vi "sib vi - cycle fail v1.vi"(0 "Amps Lo?":bool, 1 "Enable in":bool, 2 "Input Cluster":T1, 3 "SELECT":T2(ring), 4 "Amps Hi?":bool) -> (14 "(FAIL LO) out":dbl, 15 "(FAIL HI) out":dbl, 16 "(DISP) out":T3, 17 "(RESULT) out":bool, 19 "file error":errorcluster)   [LabVIEW 2013]
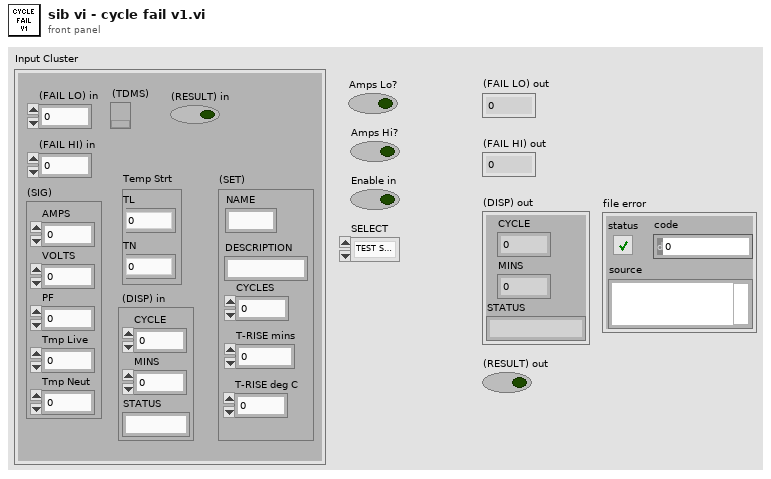
[diagram p1: front panel]
types:
  T1 = cluster{"(FAIL LO) in":dbl, "(FAIL HI) in":dbl, "(SIG)":cluster{"AMPS":dbl, "VOLTS":dbl, "PF":dbl, "Tmp Live":dbl, "Tmp Neut":dbl}, "Temp Strt":cluster{"TL":dbl, "TN":dbl}, "(SET)":cluster{"NAME":string, "DESCRIPTION":string, "CYCLES":dbl, "T-RISE mins":dbl, "T-RISE deg C":dbl}, "(TDMS)":refnum<k34>, " (DISP) in":cluster{"CYCLE":dbl, "MINS":dbl, "STATUS":string}, "(RESULT) in":bool}
  T2 = enum32{"TEST SET UP", "CYCLE TEST", "T-RISE TEST"}
  T3 = cluster{"CYCLE":dbl, "MINS":dbl, "STATUS":string}
  T4 = cluster{"AMPS":dbl, "VOLTS":dbl, "PF":dbl, "Tmp Live":dbl, "Tmp Neut":dbl}
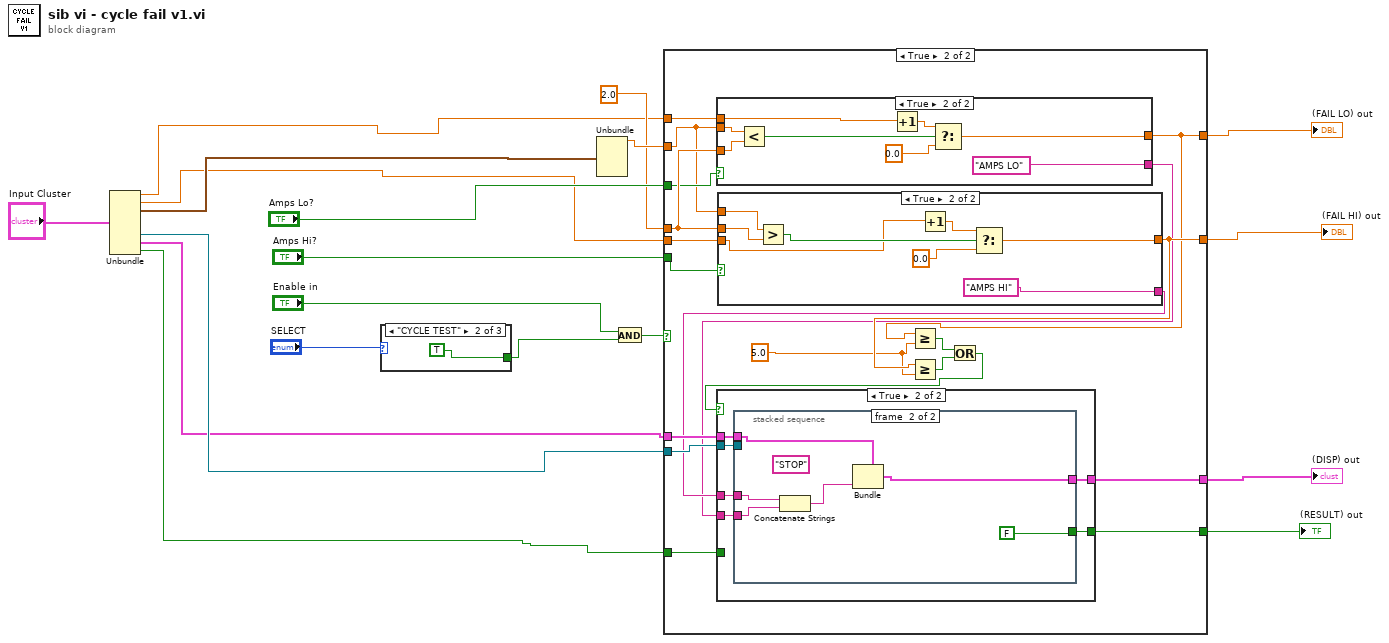
[diagram p0: block diagram]
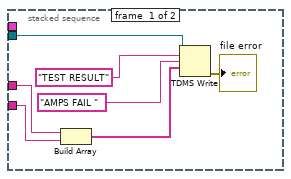
[diagram p4: hidden frame]
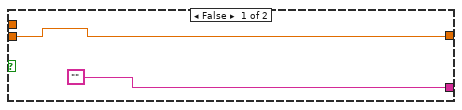
[diagram p5: hidden frame]
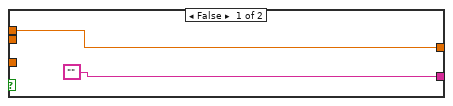
[diagram p6: hidden frame]
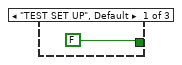
[diagram p7: hidden frame]
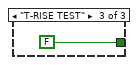
[diagram p8: hidden frame]
diagram:
  n1 = Unbundle("Input Cluster") -> ("(FAIL LO) in"=w5:dbl, "(FAIL HI) in"=w4:dbl, "(SIG)"=w7:T4, "(TDMS)"=w3:refnum<k34>, "(DISP) in"=w2:T3, "(RESULT) in"=w1:bool)  [unwired: 2 out]
  n2 = case shown="\"CYCLE TEST\"" "SELECT" {
    tunnel: [FALSE TRUE FALSE] -> w11
    frame "TEST SET UP", Default {
    }
    frame "CYCLE TEST" {
    }
    frame "T-RISE TEST" {
    }
  }
  n3 = Unbundle(w7) -> ("AMPS"=w12:dbl)  [unwired: 4 out]
  n4 = And(x="Enable in", y=w11) -> (x .and. y?=w9:bool)
  n5 = case shown="True" w9 {
    tunnel: w1 -> [w23 w45]
    tunnel: w4 -> [w25 w44]
    tunnel: [w23 w43] -> w19
    tunnel: [w24 w42] -> w18
    tunnel: w2 -> [w24 w41]
    tunnel: [w25 w40] -> w17
    tunnel: [w26 w39] -> w16
    tunnel: w5 -> [w26 w38]
    tunnel: 2.0 -> [_ w37]
    tunnel: w3 -> [_ w36]
    tunnel: "Amps Hi?" -> [_ w35]
    tunnel: "Amps Lo?" -> [_ w34]
    tunnel: w12 -> [_ w33]
    frame False {
    }
    frame True {
      w27 = 5.0
      n6 = case shown="True" w34 {
        tunnel: w33 -> [_ w86]
        tunnel: ["" "AMPS LO"] -> w31
        tunnel: w37 -> [_ w84]
        tunnel: w38 -> [w77 w80]
        tunnel: [w77 w79] -> w39
        frame False {
        }
        frame True {
          n7 = Less?(x=w86, y=w84) -> (x < y?=w83:bool)
          n8 = Increment(x=w80) -> (x+1=w82:dbl)
          n9 = Select(t=w82, s=w83, f=0.0) -> (s? t:f=w79:dbl)
        }
      }
      n10 = case shown="True" w35 {
        tunnel: w33 -> [_ w76]
        tunnel: ["" "AMPS HI"] -> w32
        tunnel: w37 -> [_ w74]
        tunnel: [w67 w70] -> w40
        tunnel: w44 -> [w67 w69]
        frame False {
        }
        frame True {
          n11 = Greater?(x=w76, y=w74) -> (0:w73:bool)
          n12 = Increment(x=w69) -> (x+1=w72:dbl)
          n13 = Select(t=w72, s=w73, f=0.0) -> (s? t:f=w70:dbl)
        }
      }
      n14 = Greater Or Equal?(x=w39, y=w27) -> (x >= y?=w30:bool)
      n15 = Greater Or Equal?(x=w40, y=w27) -> (x >= y?=w29:bool)
      n16 = Or(x=w30, y=w29) -> (x .or. y?=w28:bool)
      n17 = case shown="True" w28 {
        tunnel: w32 -> [_ w53]
        tunnel: w31 -> [_ w52]
        tunnel: w36 -> [_ w51]
        tunnel: w41 -> [w47 w50]
        tunnel: [w47 w49] -> w42
        tunnel: [w46 w48] -> w43
        tunnel: w45 -> [w46 _]
        frame False {
        }
        frame True {
          n18 = stacked-sequence {
            tunnel: w53 -> [w59 w66]
            tunnel: w52 -> [w58 w65]
            tunnel: w51 -> [w55 _]
            tunnel: w50 -> [_ w63]
            tunnel: [_ w62] -> w49
            tunnel: [_ FALSE] -> w48
            frame #0 {
              n19 = Build Array(w59, w58) -> (w57:string[])
              n20 = TDMS Write(0:w55, 5:"TEST RESULT", 7:"AMPS FAIL ", 9:w57) -> (15:→"file error":errorcluster)  [unwired: 2 in, 3 out]
            }
            frame #1 {
              (unwired) "STOP"
              n21 = Concatenate Strings(w66, w65) -> (w64:string)
              n22 = Bundle(cluster=w63, "STATUS"=w64) -> (w62:T3)  [unwired: 2 in]
            }
          }
        }
      }
    }
  }
  "(RESULT) out" <- w19
  "(DISP) out" <- w18
  "(FAIL HI) out" <- w17
  "(FAIL LO) out" <- w16
